vi "intializeCAN_EPOS+DPS.vi"(5 "DPS NodeID":u32[](array[numeric])=[7, 2], 6 "EPOS Settings":T2={"deviceName"="EPOS2", "NodeID"=8, "velocity profile"={"profileAcceleration"=1000, "profileDeceleration"=1000}}, 7 "CAN Settings":T3={"protocolStackName"="CANopen", "interfaceName"="NI_CAN 0", "portName"="CAN0", "baudrate"=500000, "timeout"=1000}) -> (0 "DPS error out":errorcluster, 1 "EPOS error out":errorcluster, 2 "ObjHandle out":T1, 3 "axis out":cluster{"keyHandle":u32, "nodeId":u16})   [LabVIEW 2019]
uses:
  <vilib>/nican/nican.llb/xobjhandle.ctl
  <vilib>/nican/nican.llb/ncNetAttr.ctl
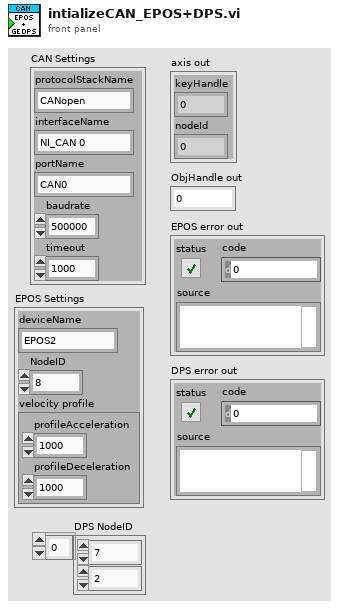
[diagram p1: front panel]
types:
  T1 = typedef "xobjhandle.ctl" = u32
  T2 = cluster{"deviceName":string, "NodeID":u8, "velocity profile":cluster{"profileAcceleration":u32, "profileDeceleration":u32}}
  T3 = cluster{"protocolStackName":string, "interfaceName":string, "portName":string, "baudrate":u32, "timeout":u32}
  T4 = typedef "ncNetAttr.ctl" = cluster{"Start On Open":enum32{"FALSE", "TRUE"}, "Baud Rate":u32, "Read Queue Length":u32, "Write Queue Length":u32, "Standard Comparator":u32, "Standard Mask":u32, "Extended Comparator":u32, "Extended Mask":u32}
  T5 = cluster{"profileAcceleration":u32, "profileDeceleration":u32}
  T6 = cluster{"deviceName":string, "protocolStackName":string, "interfaceName":string, "portName":string}
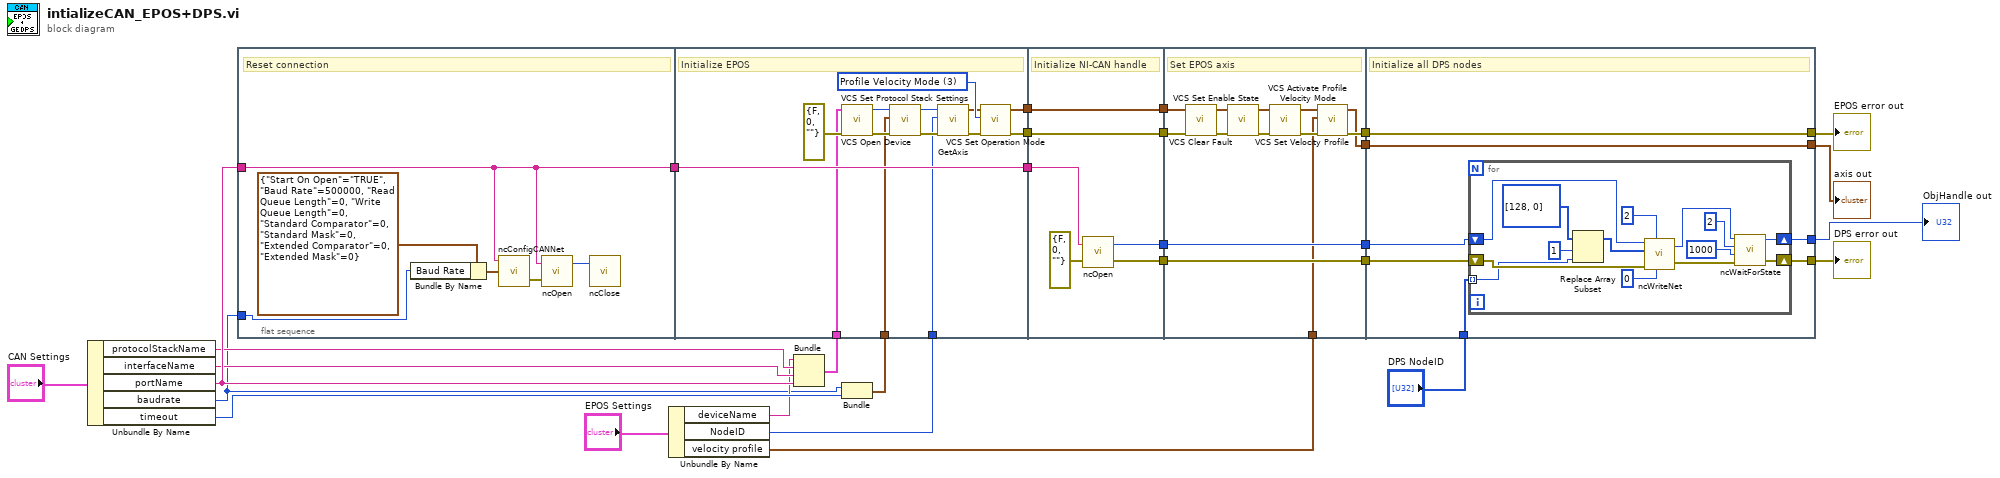
[diagram p0: block diagram]
diagram:
  n1 = Unbundle By Name("CAN Settings") -> ("protocolStackName"=w12:string, "interfaceName"=w13:string, "portName"=w17:string, "baudrate"=w1:u32, "timeout"=w15:u32)
  n2 = flat-sequence {
    tunnel: [w33] -> w29
    tunnel: w17 -> [w33]
    tunnel: w1 -> [w30]
    tunnel: [w49] -> w28
    tunnel: w29 -> [w49]
    tunnel: [w48] -> w27
    tunnel: [w47] -> w26
    tunnel: w9 -> [w38]
    tunnel: w14 -> [w37]
    tunnel: w16 -> [w36]
    tunnel: w28 -> [w54]
    tunnel: [w53] -> w25
    tunnel: [w52] -> w24
    tunnel: [w51] -> w23
    tunnel: w27 -> [w51]
    tunnel: [w50] -> w22
    tunnel: w26 -> [w50]
    tunnel: [w64] -> w21
    tunnel: [w63] -> w20
    tunnel: w25 -> [w60]
    tunnel: [w60] -> w19
    tunnel: w24 -> [w59]
    tunnel: [w59] -> w18
    tunnel: w23 -> [w58]
    tunnel: w22 -> [w57]
    tunnel: w2 -> [w56]
    tunnel: [w74] -> w3
    tunnel: [w75] -> w4
    tunnel: w21 -> [w75]
    tunnel: w20 -> [w74]
    tunnel: [w73] -> w5
    tunnel: [w72] -> w6
    tunnel: w19 -> [w71]
    tunnel: w18 -> [w70]
    tunnel: "DPS NodeID" -> [w69]
    frame #0 {
      # "Reset connection"
      n3 = Bundle By Name(cluster=T4 {"Start On Open"=enum."TRUE", "Baud Rate"=500000, "Read Queue Length"=0, "Write Queue Length"=0, "Standard Comparator"=0, "Standard Mask"=0, "Extended Comparator"=0, "Extended Mask"=0} ("CAN Network Interface Config"), "Baud Rate"=w30) -> (w31:T4)
      n4 = call <vilib>:"ncConfigCANNet.vi"("CAN Network Interface Config"=w31, "ObjName"=w33) -> ("Error out"=w34:errorcluster)  [unwired: 3 in]
      n5 = call <vilib>:"ncOpen.vi"("Error in"=w34, "ObjName"=w33) -> ("ObjHandle out"=w35:T1)  [unwired: 1 out]
      n6 = call <vilib>:"ncClose.vi"("ObjHandle in"=w35) -> ()  [unwired: 2 in, 1 out]
    }
    frame #1 {
      w45 = i8 3 items=["Profile Position Mode"=1, "Profile Velocity Mode"=3, "Homing Mode"=6, "Interpolated Position Mode"=7, "Position Mode"=-1, "Velocity Mode"=-2, "Current Mode"=-3, "Master Encoder Mode"=-5, "Step Direction Mode"=-6] ("modes of operations")
      # "Initialize EPOS"
      n7 = call <instrlib>:"VCS Open Device.vi"("error in (no error)"=errorcluster {"status"=FALSE, "code"=0, "source"=""}, "device in"=w37) -> ("error out"=w42:errorcluster, "keyHandle out"=w39:u32)  [unwired: 8 in]
      n8 = call <instrlib>:"VCS Set Protocol Stack Settings.vi"("error in (no error)"=w42, "settings"=w36, "keyHandle in"=w39) -> ("error out"=w41:errorcluster, "keyHandle out"=w40:u32)  [unwired: 7 in]
      n9 = call <instrlib>:"GetAxis.vi"("error in (no error)"=w41, "nodeId"=w38, "keyHandle in"=w40) -> ("error out"=w44:errorcluster, "axis out"=w43:cluster{"keyHandle":u32, "nodeId":u16})  [unwired: 7 in]
      n10 = call <instrlib>:"VCS Set Operation Mode.vi"("error in (no error)"=w44, "modes of operations"=w45, "axis in"=w43) -> ("error out"=w47:errorcluster, "axis out"=w48:cluster{"keyHandle":u32, "nodeId":u16})  [unwired: 7 in]
    }
    frame #2 {
      # "Initialize NI-CAN handle"
      n11 = call <vilib>:"ncOpen.vi"("Error in"=errorcluster {"status"=FALSE, "code"=0, "source"=""}, "ObjName"=w54) -> ("Error out"=w52:errorcluster, "ObjHandle out"=w53:T1)
    }
    frame #3 {
      # "Set EPOS axis"
      n12 = call <instrlib>:"VCS Clear Fault.vi"("error in (no error)"=w57, "axis in"=w58) -> ("error out"=w61:errorcluster, "axis out"=w62:cluster{"keyHandle":u32, "nodeId":u16})  [unwired: 8 in]
      n13 = call <instrlib>:"VCS Set Enable State.vi"("error in (no error)"=w61, "axis in"=w62) -> ("error out"=w66:errorcluster, "axis out"=w65:cluster{"keyHandle":u32, "nodeId":u16})  [unwired: 8 in]
      n14 = call <instrlib>:"VCS Activate Profile Velocity Mode.vi"("error in (no error)"=w66, "axis in"=w65) -> ("error out"=w67:errorcluster, "axis out"=w68:cluster{"keyHandle":u32, "nodeId":u16})  [unwired: 8 in]
      n15 = call <instrlib>:"VCS Set Velocity Profile.vi"("error in (no error)"=w67, "velocity profile"=w56, "axis in"=w68) -> ("error out"=w64:errorcluster, "axis out"=w63:cluster{"keyHandle":u32, "nodeId":u16})  [unwired: 7 in]
    }
    frame #4 {
      # "Initialize all DPS nodes"
      n16 = for {
        tunnel: w69 -> [w76] mode=indexing
        shift-right: [w79] -> w72
        shift-left: w71 -> [w78]
        shift-right: [w80] -> w73
        shift-left: w70 -> [w77]
        n17 = Replace Array Subset(array=u8[] [128, 0] ("Data"), new element=w76, index=1) -> (w89:u8[])
        n18 = call <vilib>:"ncWriteNet.vi"("ArbitrationId"=u32 0, "DataLength"=u32 2, "Error in"=w77, "Data"=w89, "ObjHandle in"=w78) -> ("Error out"=w88:errorcluster, "ObjHandle out"=w87:T1)  [unwired: 1 in]
        n19 = call <vilib>:"ncWaitForState.vi"("Error in"=w88, "Timeout"=u32 1000, "DesiredState"=u32 2, "ObjHandle in"=w87) -> ("Error out"=w80:errorcluster, "ObjHandle out"=w79:T1)  [unwired: 1 out]
      }
    }
  }
  n20 = Unbundle By Name("EPOS Settings") -> ("deviceName"=w11:string, "NodeID"=w9:u8, "velocity profile"=w2:T5)
  n21 = Bundle("deviceName"=w11, "protocolStackName"=w12, "interfaceName"=w13, "portName"=w17) -> (w14:T6)  [unwired: 1 in]
  n22 = Bundle("baudrate"=w1, "timeout"=w15) -> (w16:cluster{"baudrate":u32, "timeout":u32})  [unwired: 1 in]
  "ObjHandle out" <- w6
  "DPS error out" <- w5
  "EPOS error out" <- w4
  "axis out" <- w3
